vi "Speed_limit.vi"(1 "Speed":dbl(knob) scale=0.0..20.0) -> (0 "Speed 2":dbl)   [LabVIEW 2013]
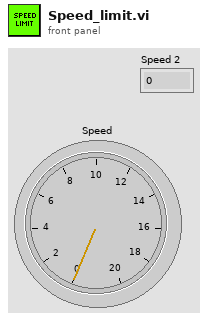
[diagram p1: front panel]
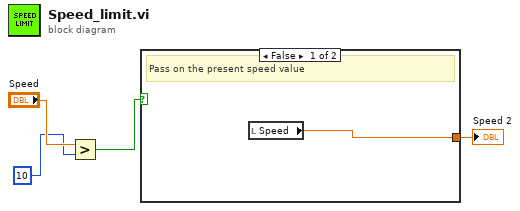
[diagram p0: block diagram]
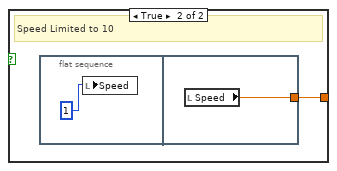
[diagram p2: hidden frame]
diagram:
  n1 = Greater?(x="Speed", y=10) -> (0:w2:bool)
  n2 = case shown="False" w2 {
    tunnel: [w5 w6] -> w4
    frame False {
      # "Pass on the present speed value"
      n3 = local read "Speed"() -> (w5:dbl)
    }
    frame True {
      # "Speed Limited to 10"
      n4 = flat-sequence {
        tunnel: [w8] -> w6
        frame #0 {
          n5 = local write "Speed"(1) -> ()
        }
        frame #1 {
          n6 = local read "Speed"() -> (w8:dbl)
        }
      }
    }
  }
  "Speed 2" <- w4
